vi "AquireShowSensorData.vi"() -> ()   [LabVIEW 2019]
panel:
  out "appended array":dbl[][](array[numeric])
  out "Smoothed data":dynamicdata(graph)
  out "Accelerometer Data":cluster{dbl, dbl, dbl}(graph)
  in  "Stop button":bool
  in  "IP Adress(IPv4)":string
  in  "Port":dbl
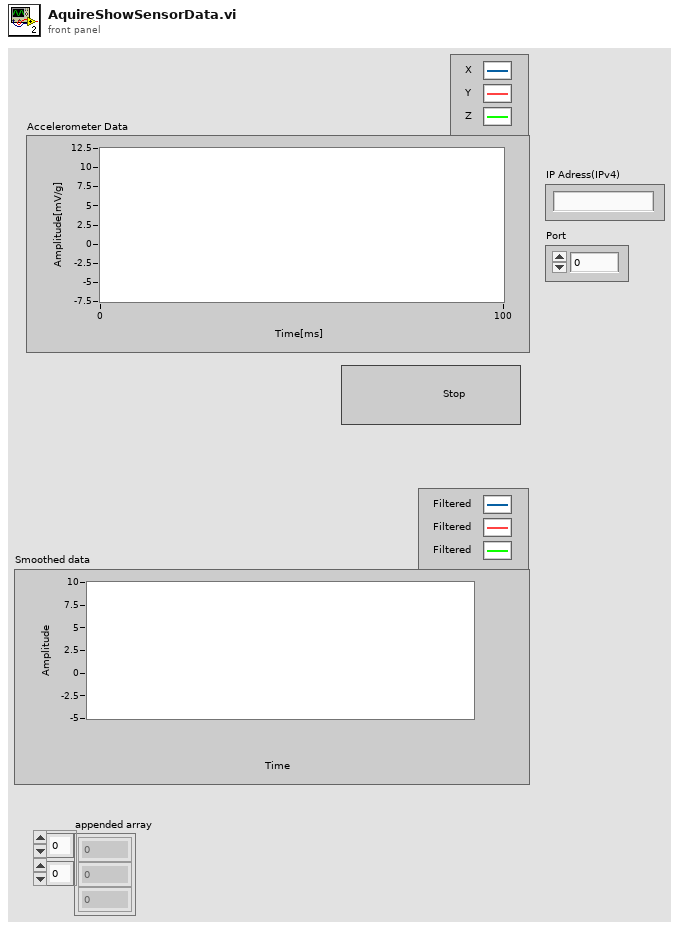
[diagram p1: front panel]
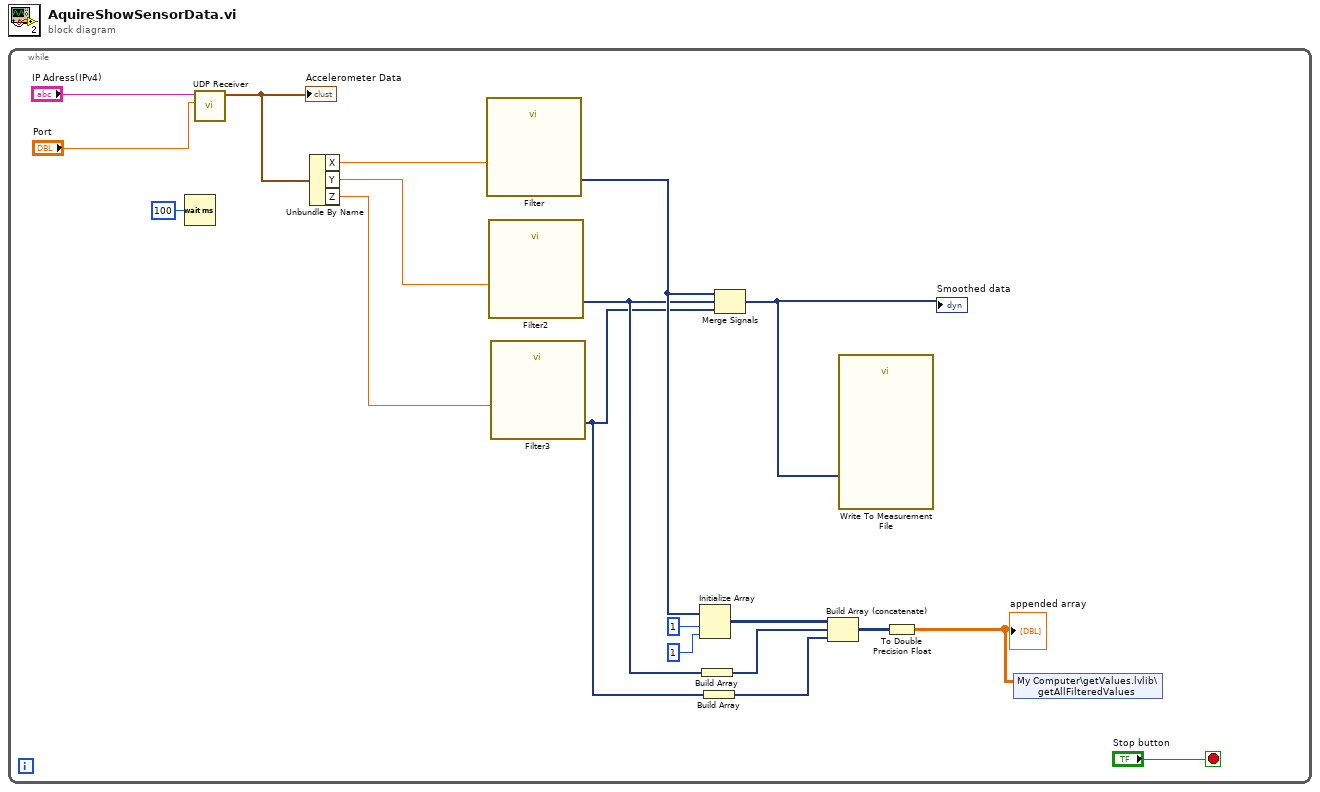
[diagram p0: block diagram]
diagram:
  n1 = while {
    stop <- "Stop button" stop-if-true
    n2 = Wait (ms)(milliseconds to wait=u32 100) -> ()  [unwired: 1 out]
    n3 = call "UDP Receiver.vi"("IP Adress"="IP Adress(IPv4)", "Port"="Port") -> ("Accelerometer Data"=w15:cluster{"X":dbl, "Y":dbl, "Z":dbl})  [unwired: 7 in, 1 out]
    "Accelerometer Data" <- w15
    n4 = Unbundle By Name(w15) -> ("X"=w14:dbl, "Y"=w13:dbl, "Z"=w12:dbl)
    n5 = call "Filter"("Signal"=w14) -> ("Filtered Signal"=w5:dynamicdata)  [unwired: 9 in, 1 out]
    n6 = call "Filter2"("Signal"=w13) -> ("Filtered Signal"=w4:dynamicdata)  [unwired: 9 in, 1 out]
    n7 = call "Filter3"("Signal"=w12) -> ("Filtered Signal"=w3:dynamicdata)  [unwired: 9 in, 1 out]
    n8 = Initialize Array(w5, 1, 1) -> (w8:dynamicdata[][])
    n9 = Build Array(w4) -> (w7:dynamicdata[])
    n10 = Build Array(w3) -> (w6:dynamicdata[])
    n11 = Merge Signals(w5, w4, w3) -> (w11:dynamicdata)
    "Smoothed data" <- w11
    n12 = Build Array (concatenate)(w8, w7, w6) -> (w2:dynamicdata[][])
    n13 = call "Write To Measurement File"("Signals"=w11) -> ()  [unwired: 16 in, 3 out]
    n14 = To Double Precision Float(number=w2) -> (double precision float=w1:dbl[][])
    "appended array" <- w1
    n15 = shared-variable "My Computer\\getValues.lvlib\\getAllFilteredValues"(w1) -> ()  [unwired: 1 in, 1 out]
  }
